vi "Add Team to Info.vi"(9 "Team Name":string, 10 "Team Number":dbl, 11 "Team Info in":T1) -> (1 "Error String":string, 2 "Team Added?":bool, 3 "Team Info out":T1)   [LabVIEW 2013]
uses:
  Team Data Array2.ctl
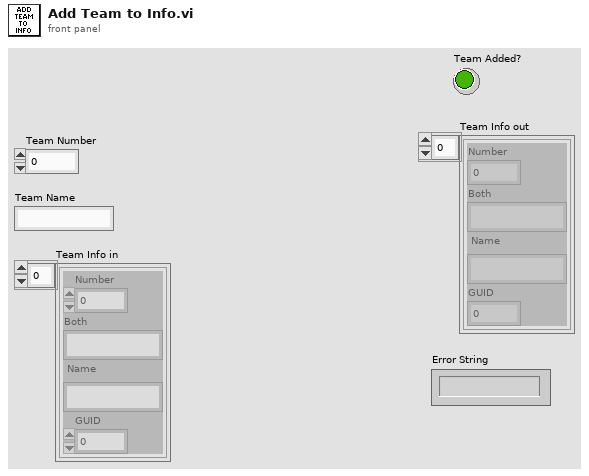
[diagram p1: front panel]
types:
  T1 = typedef "Team Data Array2.ctl" = cluster{"Number":u16, "Both":string, "Name":string, "GUID":u16}[]
  T2 = cluster{"Team Info in[0]":cluster{"Number":u16, "Both":string, "Name":string, "GUID":u16}}
  T3 = cluster{"Number":u16, "Both":string, "Name":string, "GUID":u16}
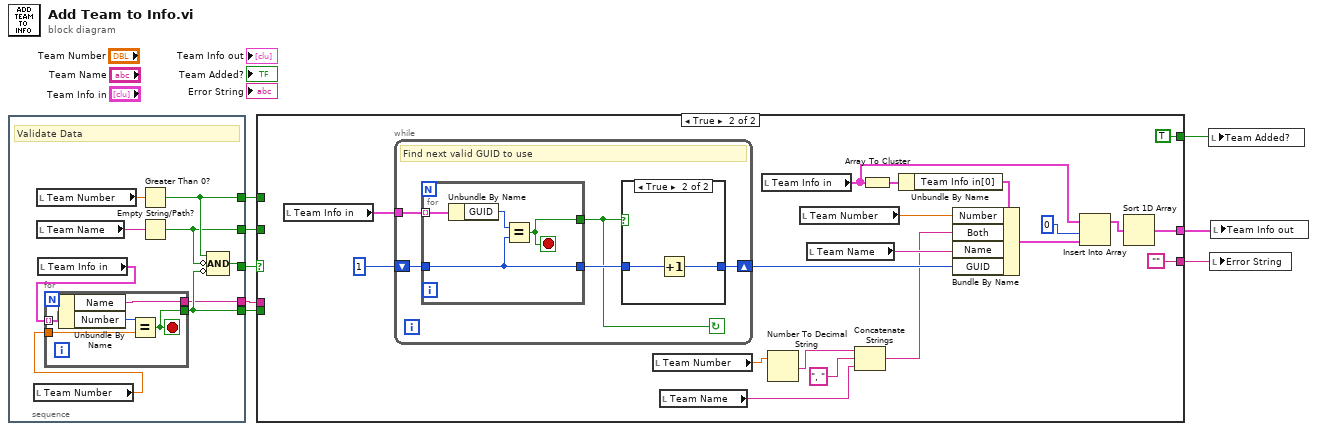
[diagram p0: block diagram]
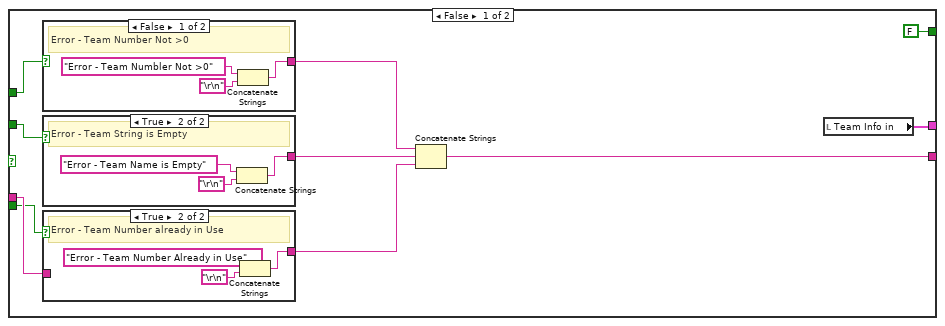
[diagram p2: hidden frame]
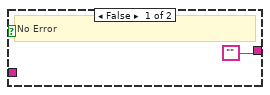
[diagram p3: hidden frame]
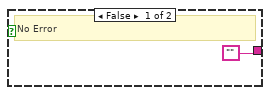
[diagram p4: hidden frame]
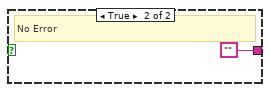
[diagram p5: hidden frame]
diagram:
  n1 = stacked-sequence {
    tunnel: [w13] -> w8
    tunnel: [w12] -> w7
    tunnel: [w11] -> w6
    tunnel: [w10] -> w5
    tunnel: [w9] -> w4
    frame #0 {
      # "Validate Data"
      n2 = local read "Team Number"() -> (w14:dbl)
      n3 = local read "Team Number"() -> (w17:dbl)
      n4 = local read "Team Name"() -> (w16:string)
      n5 = local read "Team Info in"() -> (w15:T1)
      n6 = for {
        tunnel: w15 -> [w22] mode=indexing
        tunnel: w14 -> [w20]
        tunnel: [w19] -> w10
        tunnel: [w18] -> w9
        stop <- w19 stop-if-true
        n7 = Unbundle By Name(w22) -> ("Name"=w18:string, "Number"=w21:u16)
        n8 = Equal?(x=w21, y=w20) -> (x = y?=w19:bool)
      }
      n9 = Greater Than 0?(x=w17) -> (x > 0?=w12:bool)
      n10 = Empty String/Path?(string/path=w16) -> (empty?=w11:bool)
      n11 = Compound Arithmetic op=AND(w12, invert w11, invert w10) -> (w13:bool)
    }
  }
  n12 = case shown="True" w8 {
    tunnel: [FALSE TRUE] -> w3
    tunnel: w7 -> [w31 _]
    tunnel: w6 -> [w30 _]
    tunnel: w5 -> [w28 _]
    tunnel: w4 -> [w29 _]
    tunnel: [w24 ""] -> w2
    tunnel: [w23 w45] -> w1
    frame False {
      n13 = case shown="False" w31 {
        tunnel: [w41 ""] -> w27
        frame False {
          # "Error - Team Number Not >0"
          n14 = Concatenate Strings("Error - Team Numbler Not >0", "\r\n") -> (w41:string)
        }
        frame True {
          # "No Error"
        }
      }
      n15 = case shown="True" w30 {
        tunnel: ["" w38] -> w26
        frame False {
          # "No Error"
        }
        frame True {
          # "Error - Team String is Empty"
          n16 = Concatenate Strings("Error - Team Name is Empty", "\r\n") -> (w38:string)
        }
      }
      n17 = case shown="True" w28 {
        tunnel: ["" w34] -> w25
        tunnel: w29 -> [_ _]
        frame False {
          # "No Error"
        }
        frame True {
          # "Error - Team Number already in Use"
          n18 = Concatenate Strings("Error - Team Number Already in Use", "\r\n") -> (w34:string)
        }
      }
      n19 = Concatenate Strings(w27, w26, w25) -> (w24:string)
      n20 = local read "Team Info in"() -> (w23:T1)
    }
    frame True {
      n21 = local read "Team Info in"() -> (w62:T1)
      n22 = while {
        tunnel: w62 -> [w68]
        shift-right: [w65] -> w55
        shift-left: 1 -> [w67]
        stop <- w64 continue-if-true
        # "Find next valid GUID to use"
        n23 = for {
          tunnel: w68 -> [w75] mode=indexing
          tunnel: [w73] -> w64
          tunnel: w67 -> [w72]
          tunnel: [w72] -> w66
          stop <- w73 stop-if-true
          n24 = Unbundle By Name(w75) -> ("GUID"=w74:u16)
          n25 = Equal?(x=w74, y=w72) -> (x = y?=w73:bool)
        }
        n26 = case shown="True" w64 {
          tunnel: w66 -> [w69 w71]
          tunnel: [w69 w70] -> w65
          frame False {
          }
          frame True {
            n27 = Increment(x=w71) -> (x+1=w70:i32)
          }
        }
      }
      n28 = local read "Team Number"() -> (w54:dbl)
      n29 = local read "Team Name"() -> (w51:string)
      n30 = local read "Team Info in"() -> (w49:T1)
      n31 = Number To Decimal String(number=w54) -> (decimal integer string=w52:string)  [unwired: 1 in]
      n32 = local read "Team Number"() -> (w57:dbl)
      n33 = local read "Team Name"() -> (w56:string)
      n34 = Concatenate Strings(w52, ", ", w51) -> (w50:string)
      n35 = Array To Cluster(array=w49) -> (cluster=w59:T2)
      n36 = Unbundle By Name(w59) -> ("Team Info in[0]"=w58:T3)
      n37 = Bundle By Name(cluster=w58, "Number"=w57, "Both"=w50, "Name"=w56, "GUID"=w55) -> (w48:T3)
      n38 = Insert Into Array(array=w49, index=0, new element=w48) -> (w46:T1)
      n39 = Sort 1D Array(array=w46) -> (sorted array=w45:T1)
    }
  }
  n40 = local write "Team Added?"(w3) -> ()
  n41 = local write "Error String"(w2) -> ()
  n42 = local write "Team Info out"(w1) -> ()
